vi "ZenCAM Output Template.vi"(8 "error in (no error)":errorcluster, 9 "Output Data":T1, 10 "State":string, 11 "Camera Controller in":refnum<class "Camera Controller.lvclass">) -> (0 "error out":errorcluster, 3 "Camera Controller out":refnum<class "Camera Controller.lvclass">)   [LabVIEW 2015, in "Camera Controller.lvlib" / "Camera Controller.lvclass"]
uses:
  Camera Controller.lvclass
  <vilib>/ActorFramework/Actor/Actor.lvclass
  <vilib>/vision/Image Controls.llb/IMAQ Image.ctl
  <vilib>/ActorFramework/Message Enqueuer/Message Enqueuer.lvclass
  TypeDef/Output Data.ctl
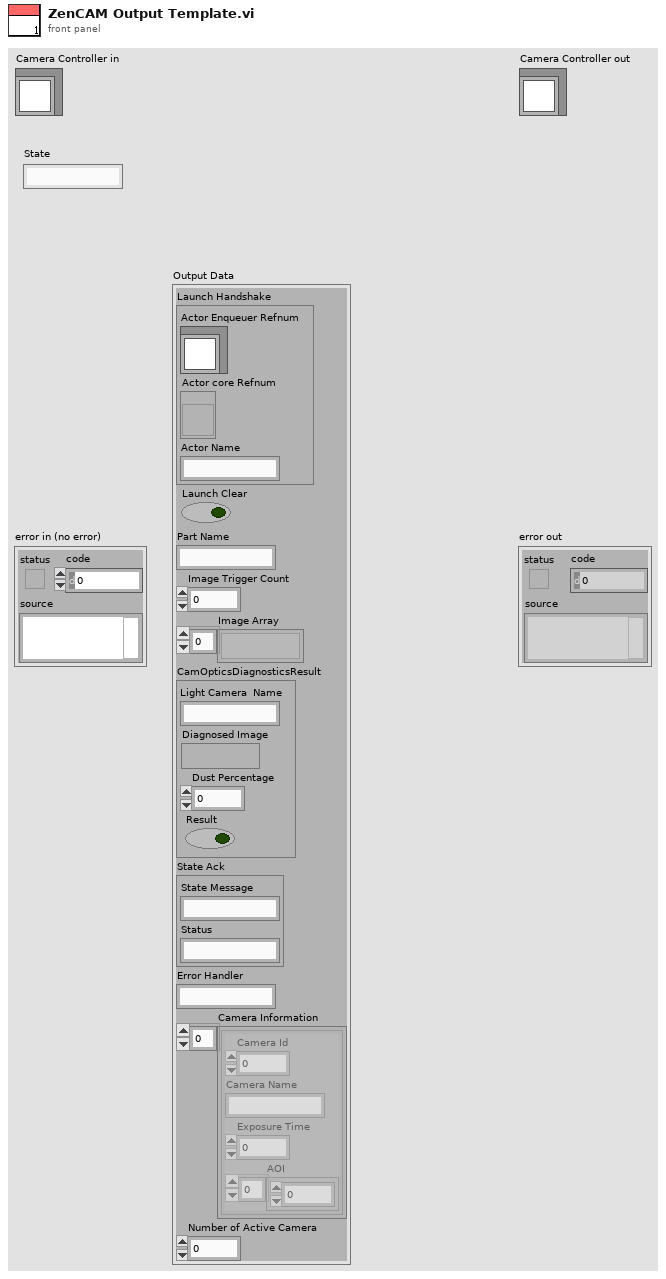
[diagram p1: front panel]
types:
  T1 = typedef "Camera Controller.lvlib/Camera Controller.lvclass/Output Data.ctl" = cluster{"Launch Handshake":cluster{"Actor Enqueuer Refnum":refnum<class "Message Enqueuer.lvclass">, "Actor core Refnum":refnum<vi>, "Actor Name":string}, "Launch Clear":bool, "Part Name":string, "Image Trigger Count":u64, "Image Array":T2[], "CamOpticsDiagnosticsResult":cluster{"Light Camera  Name":string, "Diagnosed Image":T2, "Dust Percentage":dbl, "Result":bool}, "State Ack":cluster{"State Message":string, "Status":string}, "Error Handler":string, "Camera Information":cluster{"Camera Id":i32, "Camera Name":string, "Exposure Time":i32, "AOI":i32[]}[], "Number of Active Camera":i32}
  T2 = typedef "IMAQ Image.ctl" = refnum<image>
  T3 = cluster{"Camera Names":string[], "No. of Active Cameras":u8}
  T4 = cluster{"Camera Id":i32, "Camera Name":string, "Exposure Time":i32, "AOI":i32[]}[]
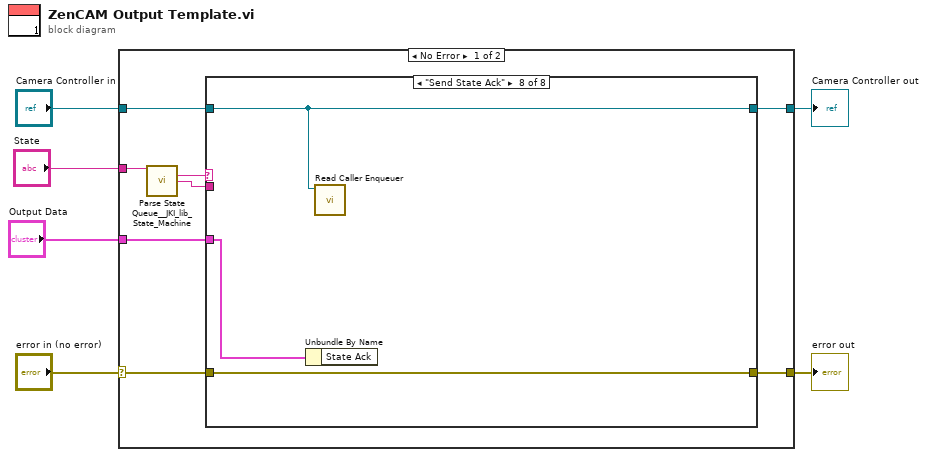
[diagram p0: block diagram]
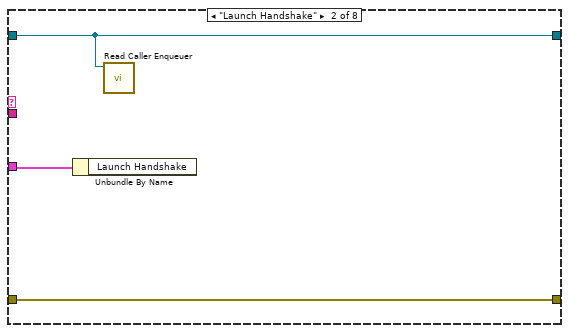
[diagram p3: hidden frame]
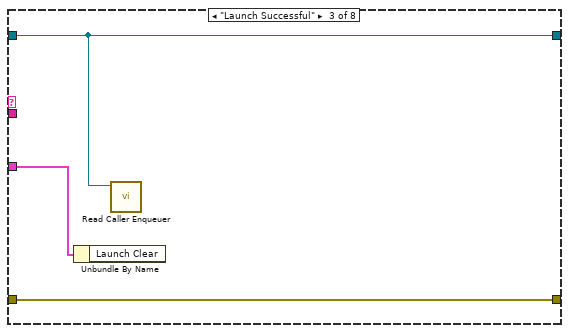
[diagram p4: hidden frame]
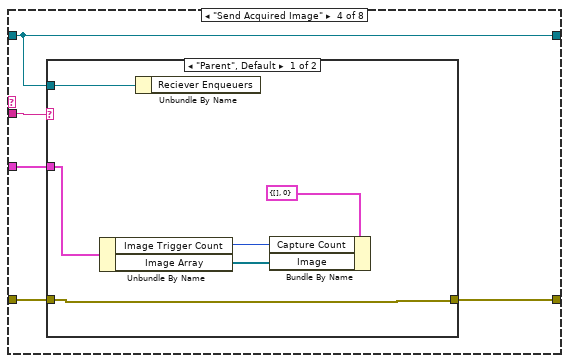
[diagram p5: hidden frame]
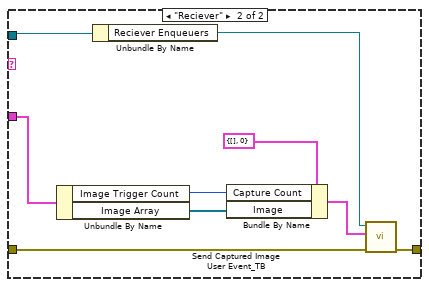
[diagram p6: hidden frame]
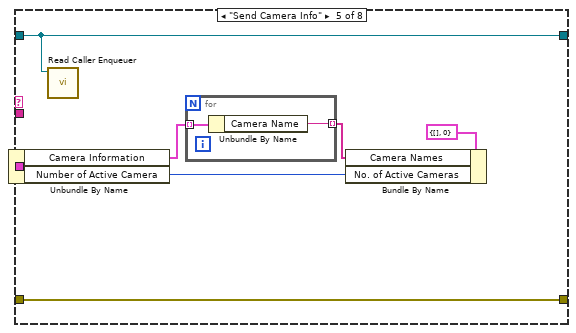
[diagram p7: hidden frame]
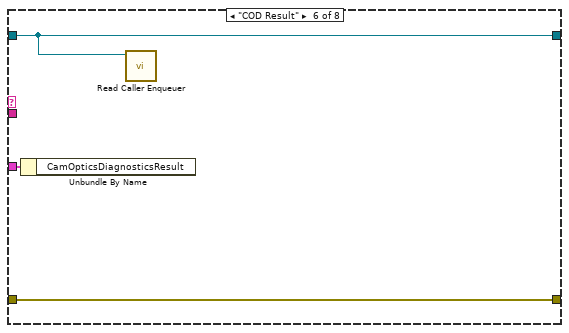
[diagram p8: hidden frame]
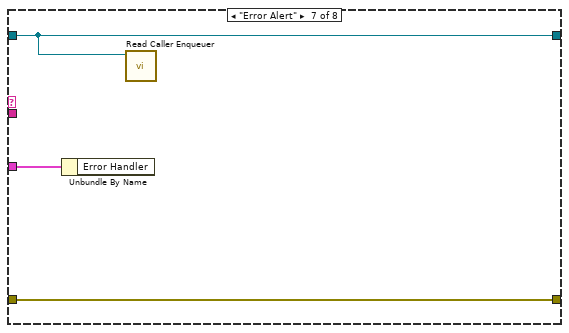
[diagram p9: hidden frame]
diagram:
  n1 = case shown="No Error" "error in (no error)" {
    selector: "error in (no error)" -> [w11 w62]
    tunnel: [w10 w62] -> w5
    tunnel: [w12 w61] -> w3
    tunnel: "Camera Controller in" -> [w13 w61]
    tunnel: "State" -> [w9 _]
    tunnel: "Output Data" -> [w14 _]
    frame No Error {
      n2 = call <vilib>:"Parse State Queue__JKI_lib_State_Machine.vi"("State Queue"=w9) -> ("Current State"=w8:string, "Arguments"=w7:string)  [unwired: 12 in, 1 out]
      n3 = case shown="\"Send State Ack\"" w8 {
        tunnel: w14 -> [_ w19 w22 w27 w49 w54 w57 w59]
        tunnel: w11 -> [w15 w17 w20 w25 w43 w52 w55 w58]
        tunnel: w13 -> [w16 w18 w21 w26 w44 w53 w56 w60]
        tunnel: [w16 w18 w21 w26 w44 w53 w56 w60] -> w12
        tunnel: [w15 w17 w20 w24 w43 w52 w55 w58] -> w10
        tunnel: w7 -> [_ _ _ w23 _ _ _ _]
        frame Default {
        }
        frame "Launch Handshake" {
          n4 = Unbundle By Name(w19) -> ()  [unwired: 1 out]
          n5 = call <vilib>:"Read Caller Enqueuer.vi"("Actor"=w18) -> ()  [unwired: 10 in, 1 out]
        }
        frame "Launch Successful" {
          n6 = Unbundle By Name(w22) -> ()  [unwired: 1 out]
          n7 = call <vilib>:"Read Caller Enqueuer.vi"("Actor"=w21) -> ()  [unwired: 10 in, 1 out]
        }
        frame "Send Acquired Image" {
          n8 = case shown="\"Parent\", Default" w23 {
            tunnel: w27 -> [w29 w42]
            tunnel: w26 -> [w30 w37]
            tunnel: w25 -> [w28 w35]
            tunnel: [w28 w34] -> w24
            frame "Parent", Default {
              n9 = Unbundle By Name(w29) -> ("Image Trigger Count"=w31:u64, "Image Array"=w32:T2[])
              n10 = Unbundle By Name(w30) -> ()  [unwired: 1 out]
              n11 = Bundle By Name(cluster=cluster{"Image":T2[], "Capture Count":u64} {"Image"=[], "Capture Count"=0} ("Captured Image"), "Capture Count"=w31, "Image"=w32) -> ()  [unwired: 1 out]
            }
            frame "Reciever" {
              n12 = Unbundle By Name(w42) -> ("Image Trigger Count"=w39:u64, "Image Array"=w40:T2[])
              n13 = Unbundle By Name(w37) -> ("Reciever Enqueuers"=w36:refnum<class "Message Enqueuer.lvclass">)
              n14 = Bundle By Name(cluster=cluster{"Image":T2[], "Capture Count":u64} {"Image"=[], "Capture Count"=0} ("Captured Image"), "Capture Count"=w39, "Image"=w40) -> (w38:cluster{"Image":T2[], "Capture Count":u64})
              n15 = call "Send Captured Image User Event_TB.vi"("error in (no error)"=w35, "Captured Image"=w38, "Message Enqueuer"=w36) -> ("error out"=w34:errorcluster)  [unwired: 7 in, 1 out]
            }
          }
        }
        frame "Send Camera Info" {
          n16 = Unbundle By Name(w49) -> ("Camera Information"=w48:T4, "Number of Active Camera"=w45:i32)
          n17 = call <vilib>:"Read Caller Enqueuer.vi"("Actor"=w44) -> ()  [unwired: 10 in, 1 out]
          n18 = for {
            tunnel: w48 -> [w51] mode=indexing
            tunnel: [w50] -> w46 mode=indexing
            n19 = Unbundle By Name(w51) -> ("Camera Name"=w50:string)
          }
          n20 = Bundle By Name(cluster=T3 {"Camera Names"=[], "No. of Active Cameras"=0} ("Camera Info"), "Camera Names"=w46, "No. of Active Cameras"=w45) -> ()  [unwired: 1 out]
        }
        frame "COD Result" {
          n21 = Unbundle By Name(w54) -> ()  [unwired: 1 out]
          n22 = call <vilib>:"Read Caller Enqueuer.vi"("Actor"=w53) -> ()  [unwired: 10 in, 1 out]
        }
        frame "Error Alert" {
          n23 = Unbundle By Name(w57) -> ()  [unwired: 1 out]
          n24 = call <vilib>:"Read Caller Enqueuer.vi"("Actor"=w56) -> ()  [unwired: 10 in, 1 out]
        }
        frame "Send State Ack" {
          n25 = Unbundle By Name(w59) -> ()  [unwired: 1 out]
          n26 = call <vilib>:"Read Caller Enqueuer.vi"("Actor"=w60) -> ()  [unwired: 10 in, 1 out]
        }
      }
    }
    frame Error {
    }
  }
  "error out" <- w5
  "Camera Controller out" <- w3
